vi "SCD30.vi"(6 "CO2 offset":dbl, 8 "error in (no error)":errorcluster, 11 "VISA resource name":refnum<visa-resource-name>) -> (0 "error out":errorcluster, 1 "Readings":T1, 2 "appended array":waveform(dbl)[](array[waveform]), 3 "VISA resource name out":refnum<visa-resource-name>)   [LabVIEW 2019]
doc: "This example performs a serial port write and a serial port read. The parameters set for the serial port must match the parameters of the connected instrument or device. The VISA Configure Serial Port VI sets the configuration parameters. The front panel displays the controls used to configure the basic parameters, such as baud rate, data bits, and parity. The VI passes the VISA resource name to other VIs that perform operations on that VISA resource. The VISA Write function sends a command to the serial device and the VISA Read function returns data based on the command. The VISA Close function then closes the reference to the serial device. It is important to close the reference; otherwise, further communication through that port might not be possible."
panel:
  out "Data Output":dbl[](array[numeric])
  # "Serial Sensor Read"
  # "(ppm)"
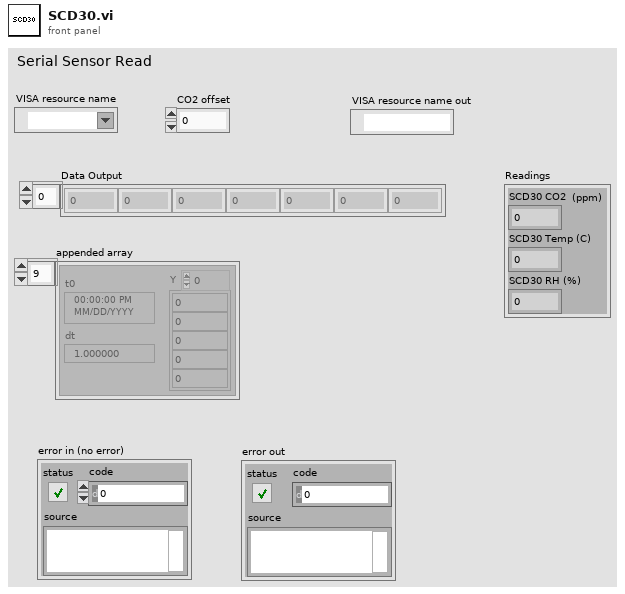
[diagram p1: front panel]
types:
  T1 = cluster{"SCD30 CO2":dbl, "SCD30 Temp (C)":dbl, "SCD30 RH (%)":dbl}
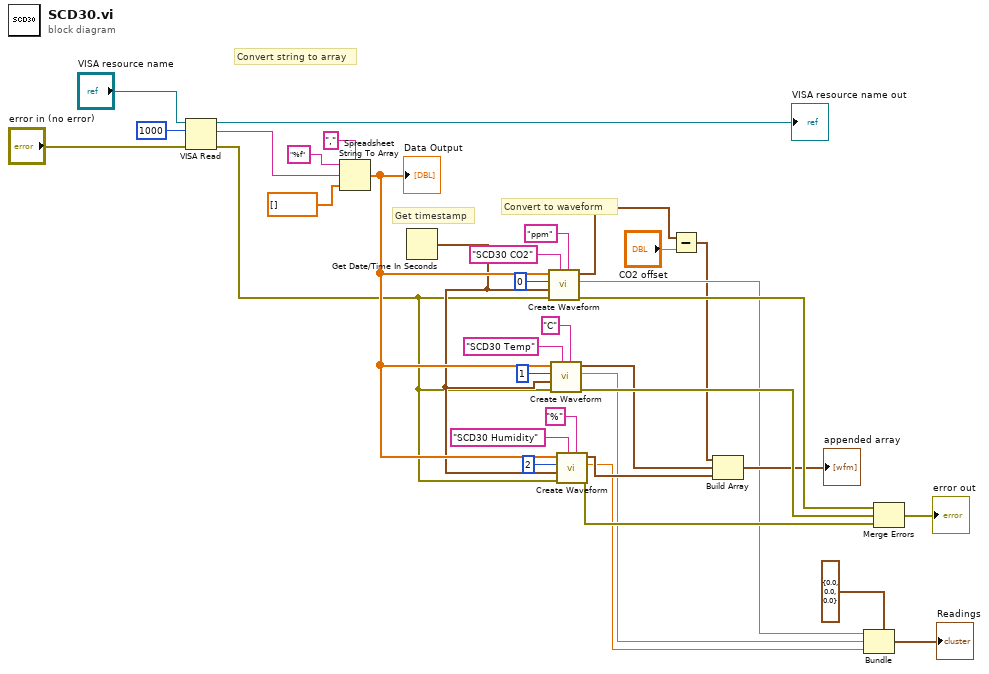
[diagram p0: block diagram]
diagram:
  # "Convert string to array"
  # "Convert to waveform"
  # "Get timestamp"
  n1 = VISA Read(VISA resource name="VISA resource name", byte count=u32 1000, error in (no error)="error in (no error)") -> (VISA resource name out=→"VISA resource name out":refnum<visa-resource-name>, read buffer=w33:string, error out=w1:errorcluster)  [unwired: 1 out]
  n2 = Spreadsheet String To Array(delimiter (Tab)=",", format string="%f", spreadsheet string=w33, array type (2D Dbl)=dbl[] []) -> (array=w14:dbl[])
  "Data Output" <- w14
  n3 = Get Date/Time In Seconds() -> (seconds since 1Jan1904=w2:timestamp)
  n4 = call "Create Waveform.vi"("Unit"="ppm", "Channel name"="SCD30 CO2", "error in (no error)"=w1, "t0"=w2, "index"=0, "array"=w14) -> ("error out"=w20:errorcluster, "Value"=w13:dbl, "output waveform"=w5:waveform(dbl))  [unwired: 3 in]
  n5 = call "Create Waveform.vi"("Unit"="C", "Channel name"="SCD30 Temp", "error in (no error)"=w1, "t0"=w2, "index"=1, "array"=w14) -> ("error out"=w19:errorcluster, "Value"=w12:dbl, "output waveform"=w17:waveform(dbl))  [unwired: 3 in]
  n6 = call "Create Waveform.vi"("Unit"="%", "Channel name"="SCD30 Humidity", "error in (no error)"=w1, "t0"=w2, "index"=2, "array"=w14) -> ("error out"=w18:errorcluster, "Value"=w11:dbl, "output waveform"=w16:waveform(dbl))  [unwired: 3 in]
  n7 = Subtract(x=w5, y="CO2 offset") -> (x-y=w4:waveform(dbl))
  n8 = Build Array(w4, w17, w16) -> (→"appended array":waveform(dbl)[])
  n9 = Bundle(cluster=cluster{"Value":dbl, "Value":dbl, "Value":dbl} {"Value"=0.0, "Value"=0.0, "Value"=0.0}, "Value"=w13, "Value"=w12, "Value"=w11) -> (→"Readings":cluster{"Value":dbl, "Value":dbl, "Value":dbl})
  n10 = Merge Errors(w20, w19, w18) -> (→"error out":errorcluster)
